vi "Heater device cluster to String.vi"(11 "Heater Device Settings":T1) -> (3 "Data to send":string="EXCT:TYPE:Unipolar:MAG:10.00:EXCT:NICK:MB1.T1:LOOP:AUX:None:PSET:1.0:HTR:None:ISET:1.0:HAUT:Manual:HSET:0.0:PIDT:Manual:DSET:1.0:TSET:0K:LVL:MB1.T1:LOOP:MAN:HVER:0:FVER:20.6:SERL:102750119:MAN:CAL:OFFS:0.0000:COLD:1.0000:INT:Linear:SCAL:1.0000:FILE:RP5.DAT:HOTL:1023.1500:CAL:TYPE:PTC:SIG:VOLT:1405.9mV:CURR:10µA:TEMP:1023.15K:POWR:14.059µW:RES:140590?:SLOP:137.409?/K:FLOW:NOT_FOUND:SIG:TEMP\n")   [LabVIEW 2019, in "Mercury iXX.lvlib" / "Heater.lvlib"]
uses:
  Heater.lvlib
  Controls/Heater Device (Set).ctl
  Controls/Heater Signals Cluster.ctl
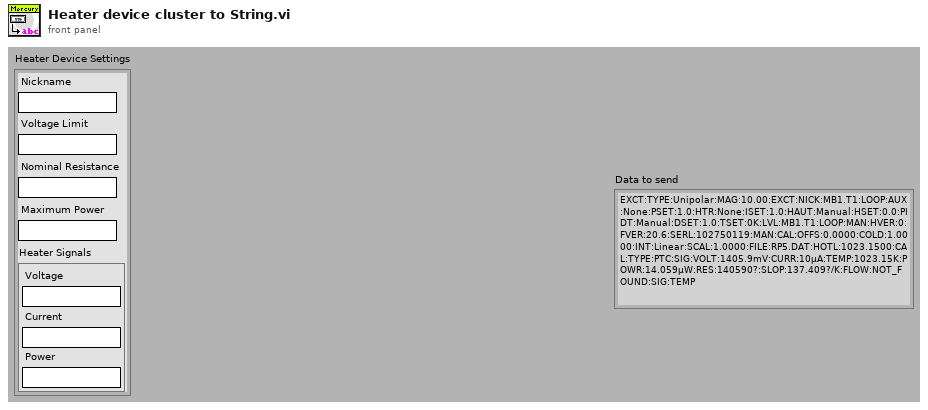
[diagram p1: front panel]
types:
  T1 = typedef "Mercury iXX.lvlib/Heater.lvlib/Heater Device (Set).ctl" = cluster{"Nickname":string, "Voltage Limit":string, "Nominal Resistance":string, "Maximum Power":string, "Heater Signals":T2}
  T2 = typedef "Mercury iXX.lvlib/Heater.lvlib/Heater Signals Cluster.ctl" = cluster{"Voltage":string, "Current":string, "Power":string}
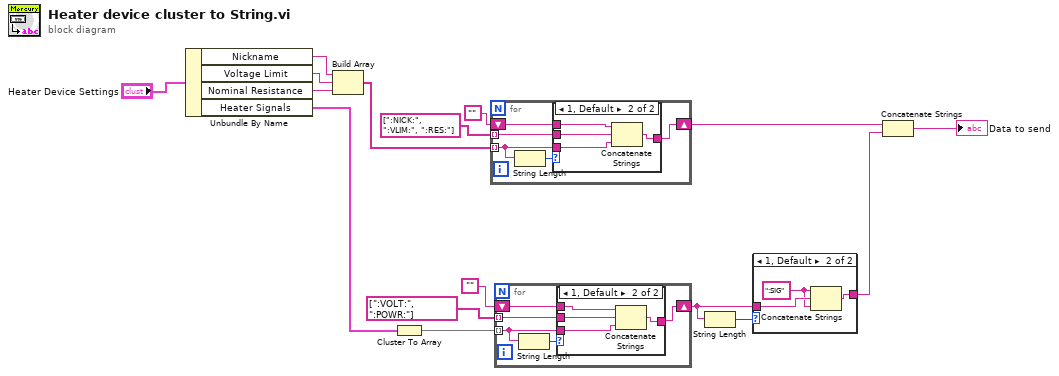
[diagram p0: block diagram]
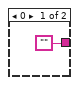
[diagram p2: hidden frame]
diagram:
  n1 = Unbundle By Name("Heater Device Settings") -> ("Nickname"=w4:string, "Voltage Limit"=w5:string, "Nominal Resistance"=w15:string, "Heater Signals"=w14:T2)
  n2 = Build Array(w4, w5, w15) -> (w3:string[])
  n3 = Cluster To Array(cluster=w14) -> (array=w10:string[])
  n4 = for {
    tunnel: w3 -> [w20] mode=indexing
    tunnel: string[] [":NICK:", ":VLIM:", ":RES:"] ("Excitation") -> [w19] mode=indexing
    shift-right: [w18] -> w6
    shift-left: "" -> [w17]
    n5 = String Length(string=w20) -> (length=w21:i32)
    n6 = case shown="1, Default" w21 {
      tunnel: w20 -> [_ w25]
      tunnel: [w22 w26] -> w18
      tunnel: w19 -> [_ w24]
      tunnel: w17 -> [w22 w23]
      frame 0 {
      }
      frame 1, Default {
        n7 = Concatenate Strings(w23, w24, w25) -> (w26:string)
      }
    }
  }
  n8 = for {
    tunnel: w10 -> [w30] mode=indexing
    tunnel: string[] [":VOLT:", ":POWR:"] ("Excitation") -> [w29] mode=indexing
    shift-right: [w27] -> w2
    shift-left: "" -> [w28]
    n9 = String Length(string=w30) -> (length=w31:i32)
    n10 = case shown="1, Default" w31 {
      tunnel: w30 -> [_ w35]
      tunnel: [w32 w36] -> w27
      tunnel: w29 -> [_ w34]
      tunnel: w28 -> [w32 w33]
      frame 0 {
      }
      frame 1, Default {
        n11 = Concatenate Strings(w33, w34, w35) -> (w36:string)
      }
    }
  }
  n12 = String Length(string=w2) -> (length=w1:i32)
  n13 = case shown="1, Default" w1 {
    tunnel: ["" w40] -> w9
    tunnel: w2 -> [_ w39]
    frame 0 {
    }
    frame 1, Default {
      w38 = ":SIG" ("string")
      n14 = Concatenate Strings(w38, w39, w38) -> (w40:string)
    }
  }
  n15 = Concatenate Strings(w6, w9) -> (→"Data to send":string)
